vi "Rectangle Comparison.vi"(9 "Second":dbl[](array[numeric]), 11 "First":dbl[](array[numeric])) -> (0 "Rect":T1, 1 "Line":T1, 3 "Scores":T2)   [LabVIEW 2018]
doc: "Compares two bounding rectangles and gives them a score based on how likely the are to be the vision target"
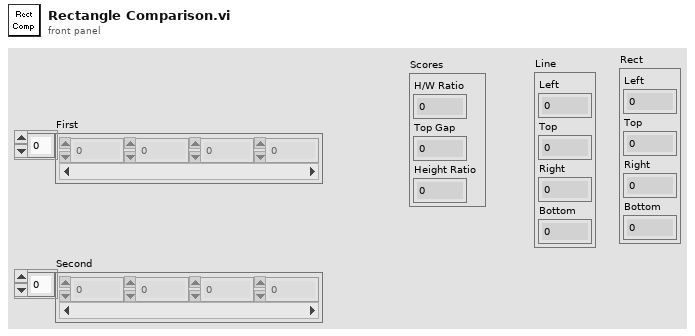
[diagram p1: front panel]
types:
  T1 = cluster{"Left":dbl, "Top":dbl, "Right":dbl, "Bottom":dbl}
  T2 = cluster{"H/W Ratio":dbl, "Top Gap":dbl, "Height Ratio":dbl}
  T3 = cluster{"[0]":dbl, "[1]":dbl, "[2]":dbl, "[3]":dbl}
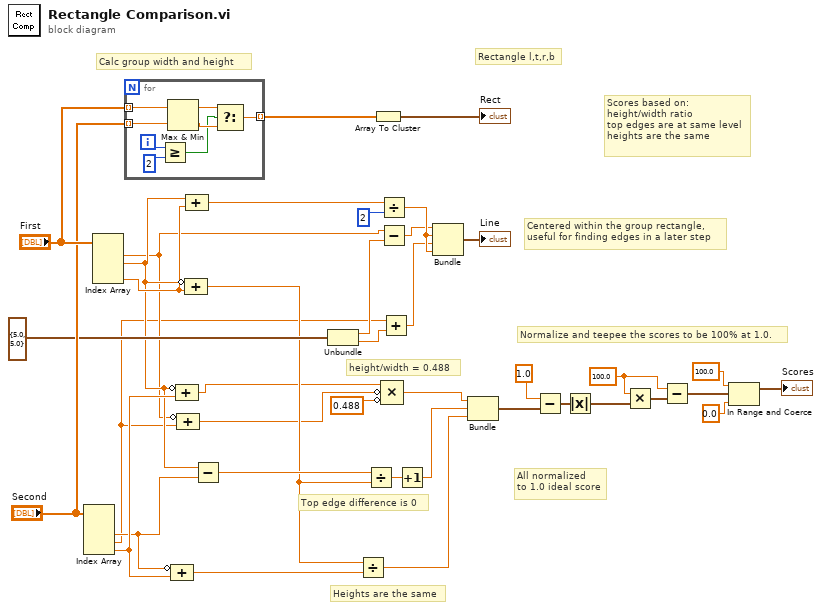
[diagram p0: block diagram]
diagram:
  w26 = 100.0 ("x/y")
  # "Scores based on:\nheight/width ratio\ntop edges are at same level\nheights are the same"
  # "height/width = 0.488"
  # "Top edge difference is 0"
  # "Heights are the same"
  # "Centered within the group rectangle,\nuseful for finding edges in a later step"
  # "All normalized\nto 1.0 ideal score"
  # "Normalize and teepee the scores to be 100% at 1.0."
  # "Calc group width and height"
  # "Rectangle l,t,r,b"
  n1 = Index Array(array="Second") -> (element #2=w9:dbl, element #3=w2:dbl, element #4=w20:dbl)  [unwired: 4 in, 1 out]
  n2 = Index Array(array="First") -> (element #1=w3:dbl, element #2=w10:dbl, element #4=w15:dbl)  [unwired: 4 in, 1 out]
  n3 = for {
    tunnel: "First" -> [w47] mode=indexing
    tunnel: "Second" -> [w46] mode=indexing
    tunnel: [w40] -> w31 mode=indexing
    i -> [w44]
    n4 = Greater Or Equal?(x=w44, y=2) -> (x >= y?=w41:bool)
    n5 = Max & Min(x=w47, y=w46) -> (max(x,y)=w43:dbl, min(x,y)=w42:dbl)
    n6 = Select(t=w43, s=w41, f=w42) -> (s? t:f=w40:dbl)
  }
  n7 = Compound Arithmetic op=ADD(invert w9, w20) -> (w11:dbl)
  n8 = Compound Arithmetic op=ADD(invert w10, w20) -> (w5:dbl)
  n9 = Compound Arithmetic op=ADD(invert w3, w2) -> (w4:dbl)
  n10 = Compound Arithmetic op=ADD(invert w10, w15) -> (w8:dbl)
  n11 = Compound Arithmetic op=ADD(w10, w15) -> (w36:dbl)
  n12 = Subtract(x=w10, y=w9) -> (x-y=w39:dbl)
  n13 = Unbundle(cluster{"Top":dbl, "Bottom":dbl} {"Top"=5.0, "Bottom"=5.0} ("Line Border")) -> ("Top"=w16:dbl, "Bottom"=w17:dbl)
  n14 = Divide(x=w8, y=w11) -> (x/y=w38:dbl)
  n15 = Divide(x=w39, y=w8) -> (x/y=w37:dbl)
  n16 = Array To Cluster(array=w31) -> (cluster=→"Rect":T3)
  n17 = Divide(x=w36, y=2) -> (x/y=w14:dbl)
  n18 = Subtract(x=w3, y=w16) -> (x-y=w13:dbl)
  n19 = Add(x=w2, y=w17) -> (x+y=w12:dbl)
  n20 = Compound Arithmetic op=MULTIPLY(w5, invert w4, invert 0.488 ("y")) -> (w6:dbl)
  n21 = Increment(x=w37) -> (x+1=w29:dbl)
  n22 = Bundle(w13, w14, w12, w14) -> (→"Line":cluster{dbl, dbl, dbl, dbl})  [unwired: 1 in]
  n23 = Bundle(w6, w29, w38) -> (w7:cluster{dbl, dbl, dbl})  [unwired: 1 in]
  n24 = Subtract(x=1.0 ("y"), y=w7) -> (x-y=w24:cluster{dbl, dbl, dbl})
  n25 = Absolute Value(x=w24) -> (abs(x)=w27:cluster{dbl, dbl, dbl})
  n26 = Multiply(x=w26, y=w27) -> (x*y=w28:cluster{dbl, dbl, dbl})
  n27 = Subtract(x=w26, y=w28) -> (x-y=w23:cluster{dbl, dbl, dbl})
  n28 = In Range and Coerce(upper limit=100.0, x=w23, lower limit=0.0) -> (coerced(x)=→"Scores":cluster{dbl, dbl, dbl})  [unwired: 1 out]
